vi "Recursion_Hanoi_zh.vi"(8 "C":string="C", 9 "B":string="B", 10 "A":string="A", 11 "Plates":u8=4) -> (3 "Step":string[](array[string]))   [LabVIEW 2012]
panel:
  out "Total_stp":i32
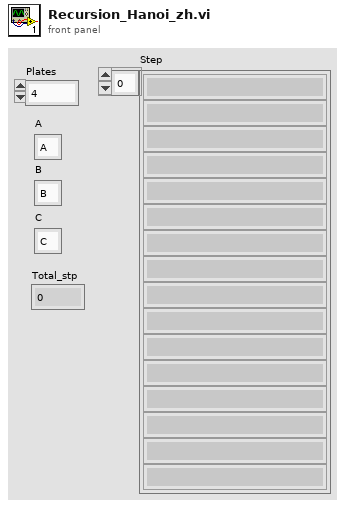
[diagram p1: front panel]
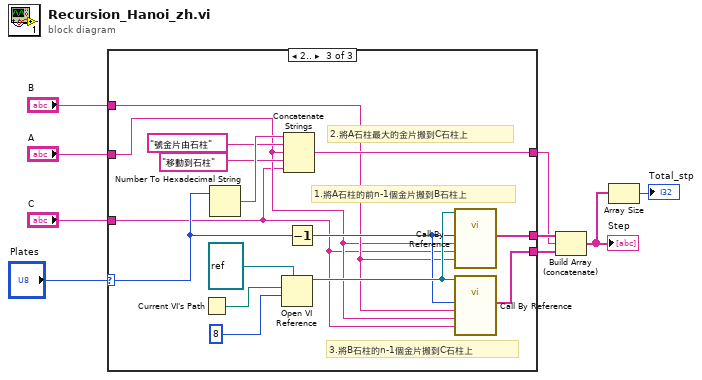
[diagram p0: block diagram]
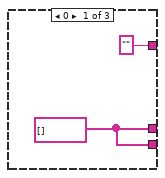
[diagram p2: hidden frame]
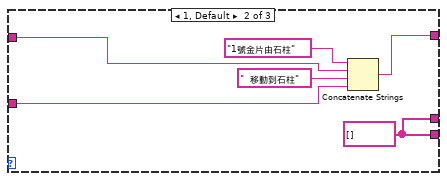
[diagram p3: hidden frame]
diagram:
  n1 = case shown="2.." "Plates" {
    selector: "Plates" -> [_ _ w29]
    tunnel: [w11 w17 w30] -> w8
    tunnel: ["" w12 w25] -> w7
    tunnel: "A" -> [_ w15 w20]
    tunnel: "C" -> [_ w13 w19]
    tunnel: [w11 w17 w22] -> w4
    tunnel: "B" -> [_ _ w21]
    frame 0 {
      w11 = string[] [] ("Array")
    }
    frame 1, Default {
      w17 = string[] [] ("Array")
      n2 = Concatenate Strings("1號金片由石柱", w15, "  移動到石柱", w13) -> (w12:string)
    }
    frame 2.. {
      # "2.將A石柱最大的金片搬到C石柱上"
      # "3.將B石柱的n-1個金片搬到C石柱上"
      # "1.將A石柱的前n-1個金片搬到B石柱上"
      n3 = Current VI's Path() -> (path=w18:path)
      n4 = Number To Hexadecimal String(2:w29) -> (0:w28:string)  [unwired: 1 in]
      n5 = Open VI Reference(type specifier VI Refnum (for type only)=refnum<vi> refnum, vi path=w18, options=8) -> (vi reference=w24:refnum<vi>)  [unwired: 3 in, 1 out]
      n6 = Concatenate Strings(w28, "號金片由石柱", w20, "移動到石柱", w19) -> (w25:string)
      n7 = Decrement(x=w29) -> (x-1=w23:u8)
      n8 = call-by-ref "?"(reference=w24, "C"=w21, "B"=w19, "A"=w20, "x (input)"=w23) -> ("Array"=w30:string[])  [unwired: 8 in, 2 out]
      n9 = call-by-ref "?"(reference=w24, "C"=w19, "B"=w20, "A"=w21, "x (input)"=w23) -> ("Array"=w22:string[])  [unwired: 8 in, 2 out]
    }
  }
  n10 = Build Array (concatenate)(w8, w7, w4) -> (w2:string[])
  "Step" <- w2
  n11 = Array Size(array=w2) -> (size(s)=→"Total_stp":i32)
